vi "I2C_ReadBlock Example.vi"(4 "length":i32=32, 5 "Bus":i32=1, 6 "Device register":u8 format="%.0x", 7 "Address":u8 format="%.0x", 8 "error in":errorcluster) -> (0 "error out":errorcluster, 3 "Block":u16[](array[numeric]) format="%.0x")   [LabVIEW 2014]
doc: "This example VI demonstrates writing a single byte to a device connected to the I2C bus."
uses:
  GPIO.lvlib
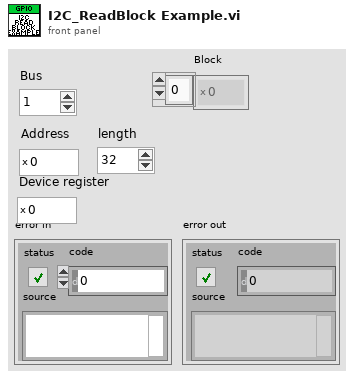
[diagram p1: front panel]
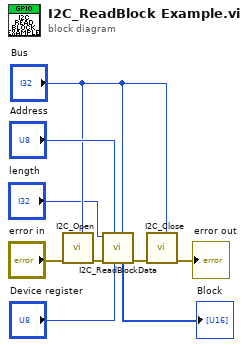
[diagram p0: block diagram]
diagram:
  n1 = call "I2C_Open.vi"("Bus"="Bus", "error in"="error in") -> ("error out"=w7:errorcluster)  [unwired: 9 in]
  n2 = call "I2C_ReadBlockData.vi"("Bus"="Bus", "Device register"="Device register", "Address"="Address", "error in"=w7, "length"="length") -> ("error out"=w6:errorcluster, "Block"=→"Block":u16[])  [unwired: 5 in]
  n3 = call "I2C_Close.vi"("Bus"="Bus", "error in"=w6) -> ("error out"=→"error out":errorcluster)  [unwired: 9 in]
